vi "PH_4_Pos_Selector.Picture MA MM1.vi"(1 "State":T1 items=["unknown", "Position I", "Position II", "Position III", "Position IV", "moving"]) -> (0 "Array MM1":picture[](array[picture]))   [LabVIEW 2014, in "PH_4_Pos_Selector.lvlib"]
uses:
  PH_4_Pos_Selector.lvlib
  PH_4_Pos_Selector.Position Selector.ctl
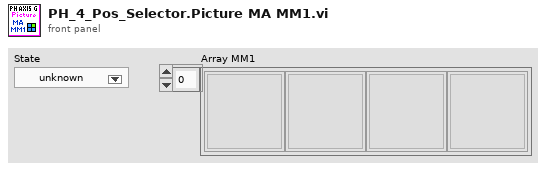
[diagram p1: front panel]
types:
  T1 = typedef "PH_4_Pos_Selector.lvlib/PH_4_Pos_Selector.Position Selector.ctl" = u16
  T2 = cluster{"left":i16, "top":i16, "right":i16, "bottom":i16}[]
  T3 = cluster{"left":i16, "top":i16, "right":i16, "bottom":i16}
  T4 = cluster{"horizontal":enum16{"left", "center", "right"}, "vertical":enum16{"top", "center", "bottom"}}
  T5 = enum16{"User-specified Font", "Application Font", "System Font", "Dialog Font"}
  T6 = cluster{"Font Name:":string, "Size":i16, "Strikeout?":bool, "Italic?":bool, "Underline?":bool, "Outline?":bool, "Shadow?":bool, "Bold?":bool}
  T7 = cluster{"Width":u16, "Style":enum32{"Solid", "Dash", "Dot", "DashDot", "DashDotDot"}}
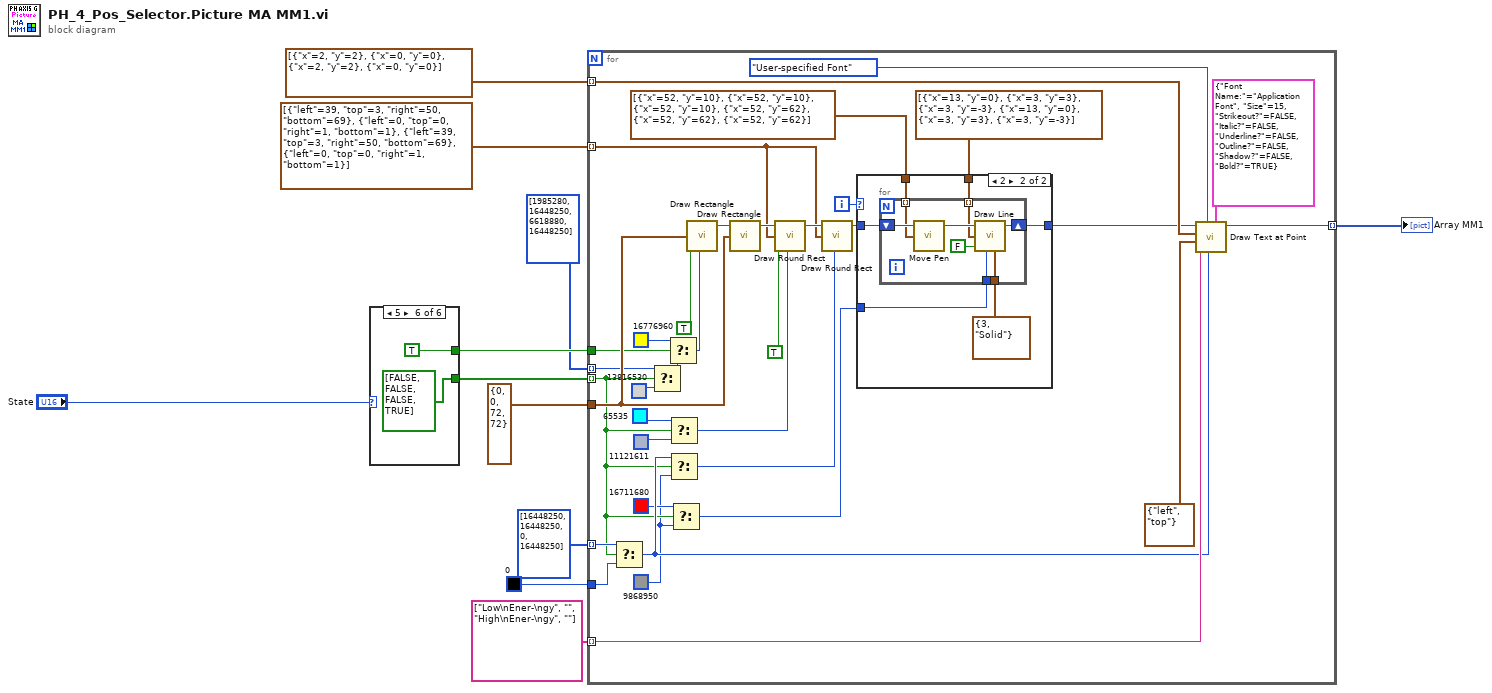
[diagram p0: block diagram]
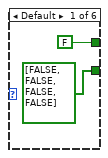
[diagram p2: hidden frame]
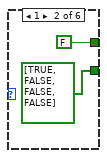
[diagram p3: hidden frame]
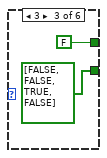
[diagram p4: hidden frame]
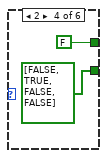
[diagram p5: hidden frame]
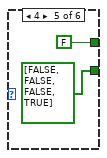
[diagram p6: hidden frame]
diagram:
  n1 = case shown="5" "State" {
    tunnel: [bool[] [FALSE, FALSE, FALSE, FALSE] bool[] [TRUE, FALSE, FALSE, FALSE] bool[] [FALSE, FALSE, TRUE, FALSE] bool[] [FALSE, TRUE, FALSE, FALSE] bool[] [FALSE, FALSE, FALSE, TRUE] bool[] [FALSE, FALSE, FALSE, TRUE]] -> w9
    tunnel: [FALSE FALSE FALSE FALSE FALSE TRUE] -> w8
    frame Default {
    }
    frame 1 {
    }
    frame 3 {
    }
    frame 2 {
    }
    frame 4 {
    }
    frame 5 {
    }
  }
  n2 = for {
    tunnel: T3 {"left"=0, "top"=0, "right"=72, "bottom"=72} ("rect") -> [w57]
    tunnel: w9 -> [w30] mode=indexing
    tunnel: w8 -> [w54]
    tunnel: [w48] -> w11 mode=indexing
    tunnel: string[] ["Low\nEner-\ngy", "", "High\nEner-\ngy", ""] -> [w49] mode=indexing
    tunnel: u32[] [1985280, 16448250, 6618880, 16448250] -> [w47] mode=indexing
    tunnel: u32[] [16448250, 16448250, 0, 16448250] -> [w46] mode=indexing
    tunnel: u32 0 -> [w45]
    tunnel: cluster{"x":i16, "y":i16}[] [{"x"=2, "y"=2}, {"x"=0, "y"=0}, {"x"=2, "y"=2}, {"x"=0, "y"=0}] -> [w34] mode=indexing
    tunnel: T2 [{"left"=39, "top"=3, "right"=50, "bottom"=69}, {"left"=0, "top"=0, "right"=1, "bottom"=1}, {"left"=39, "top"=3, "right"=50, "bottom"=69}, {"left"=0, "top"=0, "right"=1, "bottom"=1}] -> [w35] mode=indexing
    i -> [w26]
    w29 = u32 9868950
    n3 = Select(t=w46, s=w30, f=w45) -> (s? t:f=w37:u32)
    n4 = Select(t=w47, s=w30, f=u32 13816530) -> (s? t:f=w52:u32)
    n5 = Select(t=u32 16776960, s=w54, f=w52) -> (s? t:f=w51:u32)
    n6 = Select(t=u32 65535 ("color(black)"), s=w30, f=u32 11121611) -> (s? t:f=w39:u32)
    n7 = Select(t=w37, s=w30, f=w29) -> (s? t:f=w36:u32)
    n8 = Select(t=u32 16711680 ("color(black)"), s=w30, f=w29) -> (s? t:f=w28:u32)
    n9 = call <vilib>:"Draw Rectangle.vi"("rect"=w57, "fill?(F)"=TRUE, "color(black)"=w51) -> ("new picture"=w58:picture)  [unwired: 6 in]
    n10 = call <vilib>:"Draw Rectangle.vi"("picture"=w58, "rect"=w57) -> ("new picture"=w43:picture)  [unwired: 7 in]
    n11 = call <vilib>:"Draw Round Rect.vi"("picture"=w43, "rect"=w35, "fill?(F)"=TRUE, "color(black)"=w39) -> ("new picture"=w42:picture)  [unwired: 5 in]
    n12 = call <vilib>:"Draw Round Rect.vi"("picture"=w42, "rect"=w35, "color(black)"=w36) -> ("new picture"=w27:picture)  [unwired: 6 in]
    n13 = case shown="2" w26 {
      tunnel: [w59 w65] -> w32
      tunnel: w28 -> [_ w64]
      tunnel: w27 -> [w59 w62]
      tunnel: cluster{"x":i16, "y":i16}[] [{"x"=52, "y"=10}, {"x"=52, "y"=10}, {"x"=52, "y"=10}, {"x"=52, "y"=62}, {"x"=52, "y"=62}, {"x"=52, "y"=62}] -> [_ w61]
      tunnel: cluster{"x":i16, "y":i16}[] [{"x"=13, "y"=0}, {"x"=3, "y"=3}, {"x"=3, "y"=-3}, {"x"=13, "y"=0}, {"x"=3, "y"=3}, {"x"=3, "y"=-3}] -> [_ w60]
      frame Default {
      }
      frame 2 {
        n14 = for {
          tunnel: w64 -> [w72]
          tunnel: T7 {"Width"=3, "Style"=enum."Solid"} ("pen") -> [w71]
          tunnel: w61 -> [w67] mode=indexing
          shift-right: [w73] -> w65
          shift-left: w62 -> [w70]
          tunnel: w60 -> [w66] mode=indexing
          n15 = call <vilib>:"Move Pen.vi"("new position"=w67, "picture"=w70) -> ("new picture"=w69:picture)  [unwired: 3 in]
          n16 = call <vilib>:"Draw Line.vi"("picture"=w69, "end point"=w66, "absolute coordinates?(T)"=FALSE, "color(black)"=w72, "pen"=w71) -> ("new picture"=w73:picture)  [unwired: 4 in]
        }
      }
    }
    n17 = call <vilib>:"Draw Text at Point.vi"("[user-specified font]"=T6 {"Font Name:"="Application Font", "Size"=15, "Strikeout?"=FALSE, "Italic?"=FALSE, "Underline?"=FALSE, "Outline?"=FALSE, "Shadow?"=FALSE, "Bold?"=TRUE}, "text color(black)"=w37, "desired font(Application)"=T5."User-specified Font", "text"=w49, "alignment(left, top)"=T4 {"horizontal"=enum."left", "vertical"=enum."top"}, "origin"=w34, "picture"=w32) -> ("new picture"=w48:picture)  [unwired: 3 in, 1 out]
  }
  "Array MM1" <- w11
